vi "Initialize.vi"(8 "error in (no error)":errorcluster, 11 "Component Configuration in":refnum<class "Component Configuration.lvclass">) -> (0 "error out":errorcluster, 3 "Component Configuration out":refnum<class "Component Configuration.lvclass">)   [LabVIEW 2017, in "DSF Core.lvlib" / "Component Configuration.lvclass"]
uses:
  Component Configuration.lvclass
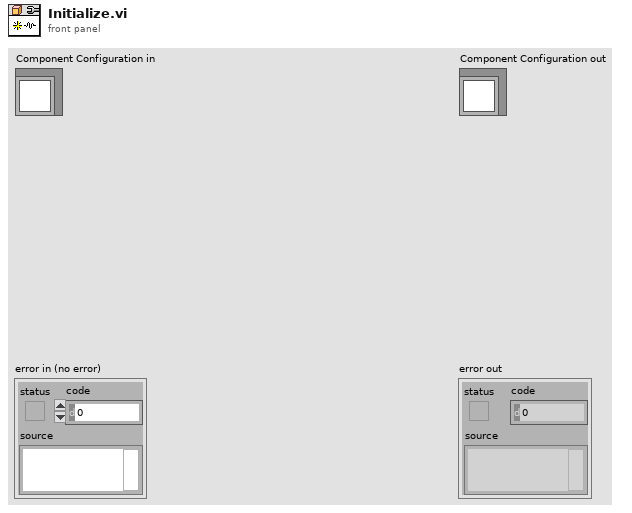
[diagram p1: front panel]
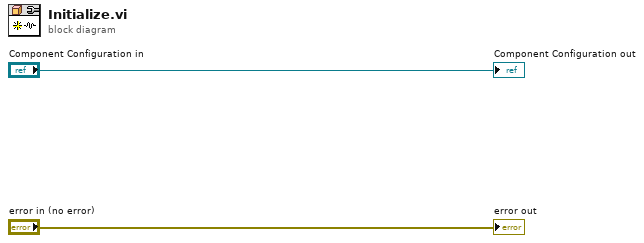
[diagram p0: block diagram]
diagram:
  "error out" <- "error in (no error)"
  "Component Configuration out" <- "Component Configuration in"
